vi "Form Single Group.vi"(8 "error in (no error)":errorcluster, 10 "Names":string[](array[string]), 11 "Group":string) -> (0 "error out":errorcluster)   [LabVIEW 2010, in "Current Value Table.lvlib"]
uses:
  Current Value Table.lvlib
  FGVs/Group Memory Methods.ctl
  FGVs/Tag Memory Methods.ctl
  Errors/Generate Error.vi
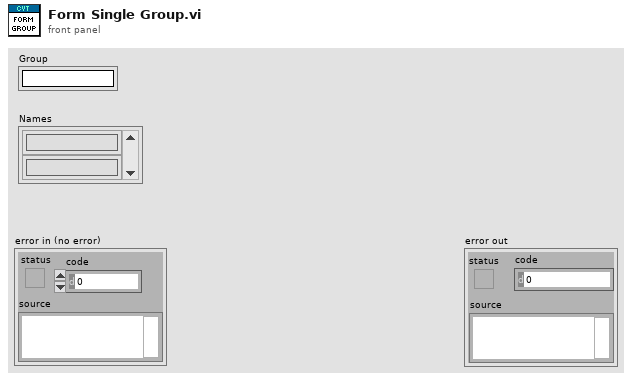
[diagram p1: front panel]
types:
  T1 = typedef "Current Value Table.lvlib/Group Memory Methods.ctl" = enum16{"Clear", "Read Indices in Group", "List Groups", "List Tags by Type", "List Tags", "Delete Group", "Check Group Existence", "Create Group"}
  T2 = typedef "Current Value Table.lvlib/Tag Memory Methods.ctl" = enum16{"Clear", "Read Tag Index", "Read Tag Indices", "Generate Group", "Add Tag", "Overwrite Tag", "Read Description", "Get Stored Tags"}
  T3 = typedef "Current Value Table.lvlib/Index Types.ctl" = cluster{"Data Type":T4, "Index":i32}
  T4 = typedef "Current Value Table.lvlib/Data Types.ctl" = enum16{"Double", "Single", "I64", "I32", "I16", "I8", "U64", "U32", "U16", "U8", "String", "Boolean", "Array of U8", "Array of U16", "Array of U32", "Array of U64", "Array of I64", "Array of I32", "Array of I16", "Array of I8", "Array of Double", "Array of Single", "Array of Boolean", "Array of String"}
  T5 = typedef "Current Value Table.lvlib/Group Initialization set.ctl" = cluster{"Index-Type Set":T6, "Tags":string[]}
  T6 = typedef "Current Value Table.lvlib/Typed Index Set.ctl" = cluster{"Data Type":T4, "Indices":i32[]}
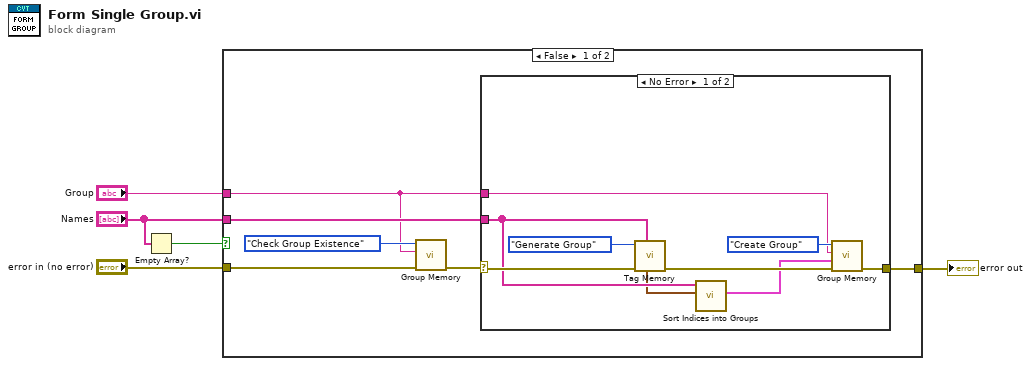
[diagram p0: block diagram]
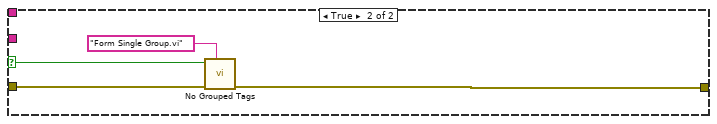
[diagram p3: hidden frame]
diagram:
  n1 = Empty Array?(array="Names") -> (empty?=w2:bool)
  n2 = case shown="False" w2 {
    selector: w2 -> [_ w23]
    tunnel: "Group" -> [w8 _]
    tunnel: "Names" -> [w9 _]
    tunnel: [w7 w24] -> w4
    tunnel: "error in (no error)" -> [w6 w25]
    frame False {
      n3 = call "Group Memory.vi"("error in (no error)"=w6, "Group"=w8, "Method"=Group_Memory_Methods."Check Group Existence") -> ("error out"=w10:errorcluster)  [unwired: 5 in, 3 out]
      n4 = case shown="No Error" w10 {
        selector: w10 -> [w20 w21]
        tunnel: w9 -> [w13 _]
        tunnel: w8 -> [w15 _]
        tunnel: [w14 w21] -> w7
        frame No Error {
          n5 = call "Tag Memory.vi"("Tags"=w13, "error in (no error)"=w20, "Method"=Tag_Memory_Methods."Generate Group") -> ("error out"=w18:errorcluster, "Group Indices Out"=w12:T3[])  [unwired: 3 in, 4 out]
          n6 = call "Sort Indices into Groups.vi"("Indices To Add"=w12, "Tags"=w13) -> ("Group Initialization Set"=w17:T5[])  [unwired: 9 in]
          n7 = call "Group Memory.vi"("error in (no error)"=w18, "Group Initialization Set"=w17, "Group"=w15, "Method"=Group_Memory_Methods."Create Group") -> ("error out"=w14:errorcluster)  [unwired: 4 in, 3 out]
        }
        frame Error {
        }
      }
    }
    frame True {
      n8 = call "No Grouped Tags.vi"("caller name"="Form Single Group.vi", "error in (no error)"=w25, "Empty List?"=w23) -> ("error out"=w24:errorcluster)  [unwired: 8 in]
    }
  }
  "error out" <- w4
